vi "Sort Fcurve wfms.vi"(0 "reference in":refnum<class "Fcurve.lvclass">, 1 "Channels In":waveform(dbl)[](array[waveform]), 5 "error in (no error)":errorcluster) -> (7 "Fcurve out":cluster{"X":dbl[], "Y":dbl[]}[](graph), 14 "reference out":refnum<class "Fcurve.lvclass">, 19 "error out":errorcluster)   [LabVIEW 2019, in "Fcurve.lvclass"]
doc: "Sorts wfms into Fcurve. [0] Deflection, [1] Zposition"
uses:
  Fcurve.lvclass
  TDMS_DataHandler_class/property name combo box.ctl
  TDMS_DataHandler_class/TDMS_DataHandler.lvclass
panel:
  out "contact point index out":i32
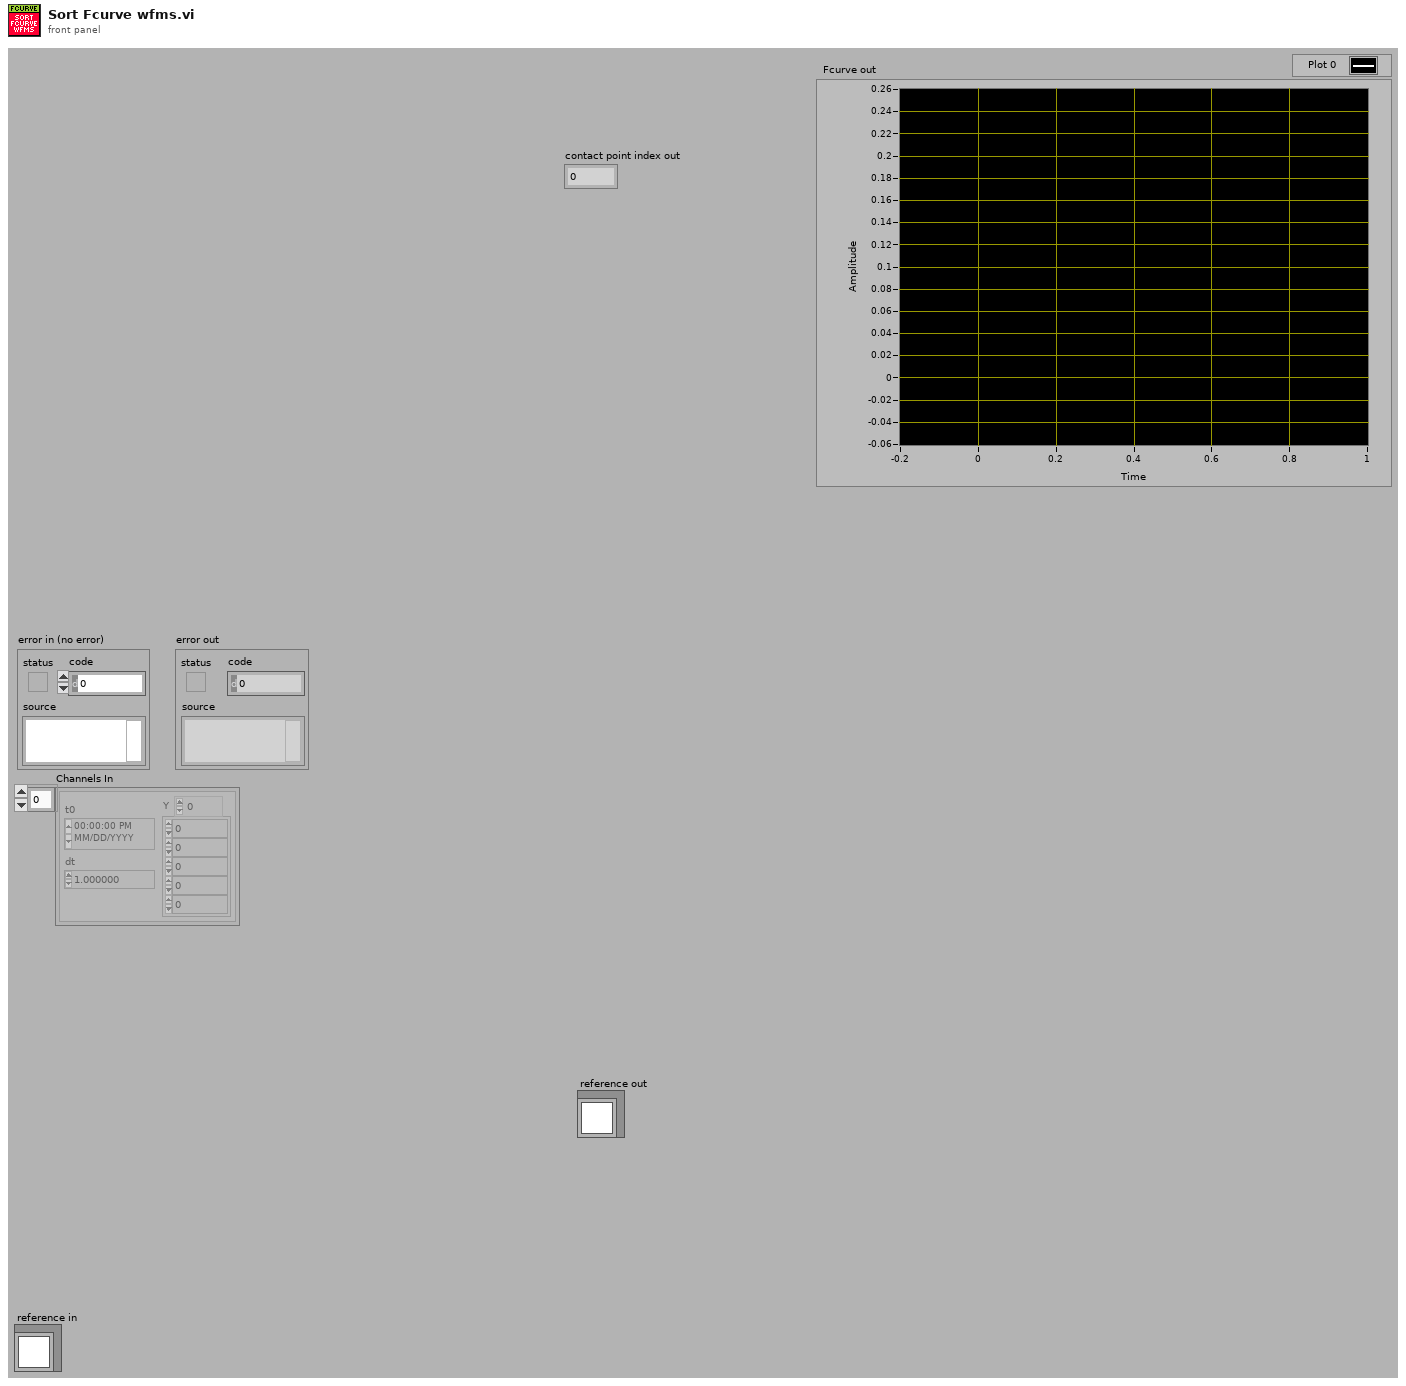
[diagram p1: front panel]
types:
  T1 = typedef "TDMS_DataHandler.lvclass/property name combo box.ctl" = string
  T2 = typedef "Fcurve.lvclass/ObjectAttributes.ctl" = cluster{"MyAttribute":dbl, "Fcurve Metadata":T3, "Contact Spread of dev":dbl, "Tau Delay (ms)":dbl, "Points of contact":dbl, "Def_wfm":cluster{"Max":dbl, "Min":dbl}, "Zpos_wfm":cluster{"Max":dbl, "Min":dbl}, "Contact stat?":bool, "Real AI dt (s)":dbl, "Decimation":cluster{"App":cluster{"Dec":i32, "apply":bool}, "Con":cluster{"Dec":i32, "apply":bool}, "Ret":cluster{"Dec":i32, "apply":bool}}, "Segment def[0]":dbl, "Segment Zpos[0]":dbl, "Raw Datum":waveform(dbl)[], "Group metadata":T4, "M_data obj":refnum<class "metadata.lvclass">, "Channel name(s)":string[], "Segment fcurve data":cluster{"X":dbl[], "Y":dbl[]}[], "Segment duration":cluster{"Start":i32, "Duration":i32}[], "Segment info":T5[], "Segment durations (S)":dbl[], "Segments Maxmin":T7[]}
  T3 = typedef "Fcurve.lvclass/Metadata.ctl" = cluster{"dt (us)":dbl, "Dec Factor":dbl, "Z piezo Sensitivity (nm/V)":dbl, "K (N/m)":dbl, "Sp (V)":dbl, "Contact (ms)":dbl, "Zpos contact":dbl, "Vel_app (nm/s)":dbl, "Vel_ret (nm/s)":dbl, "deltaV (nm)":dbl, "Def_V0 (v)":dbl, "Piezo gain":dbl, "invOLS (nm/V)":dbl}
  T4 = typedef "TDMS_DataHandler.lvclass/Fcurve Meta data.ctl" = cluster{"property names":string[], "property values":variant[]}
  T5 = typedef "Fcurve.lvclass/Fcurve segments --cluster.ctl" = cluster{"type":T6, "nb points":i32, "dec factor":u32, "sampling rate (S/s)":u32}
  T6 = typedef "metadata.lvclass/Segment type--combobox.ctl" = string
  T7 = typedef "Fcurve.lvclass/Segment MaxMin --cluster.ctl" = cluster{"Def":cluster{"max value":dbl, "min value":dbl}, "Zpos":cluster{"max value":dbl, "min value":dbl}}
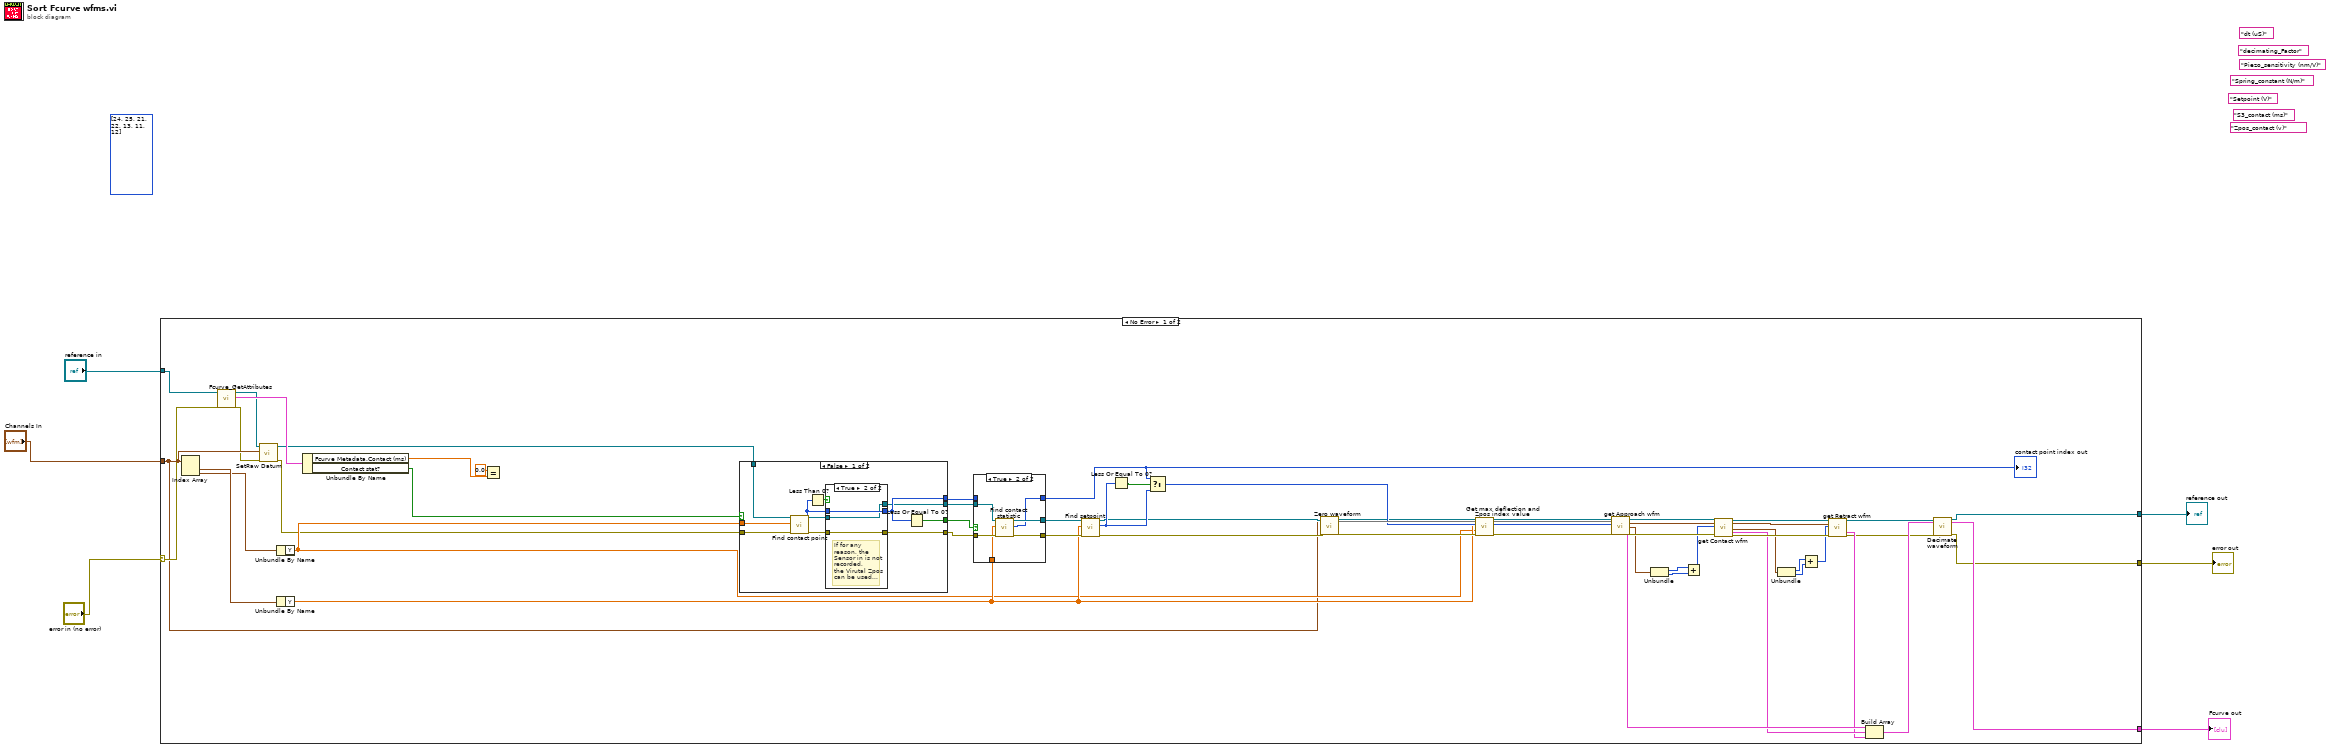
[diagram p0: block diagram]
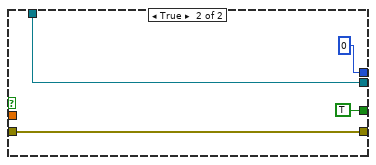
[diagram p3: hidden frame]
diagram:
  (unwired) i32[] [24, 25, 21, 22, 13, 11, 12] ("Array")
  (unwired) T1 "Setpoint (V)" ("Combo Box")
  (unwired) T1 "S3_contact (ms)" ("Combo Box")
  (unwired) T1 "Zpos_contact (v)" ("Combo Box")
  (unwired) T1 "Spring_constant (N/m)" ("Combo Box")
  (unwired) T1 "Piezo_sensitivity (nm/V)" ("Combo Box")
  (unwired) T1 "decimating_Factor" ("Combo Box")
  (unwired) T1 "dt (uS)" ("Combo Box")
  n1 = case shown="No Error" "error in (no error)" {
    selector: "error in (no error)" -> [w26 w92]
    tunnel: "reference in" -> [w59 w93]
    tunnel: [w21 w93] -> w5
    tunnel: [w18 w92] -> w4
    tunnel: [w23 _] -> w2
    tunnel: "Channels In" -> [w11 _]
    frame No Error {
      n2 = Index Array(array=w11) -> (element #1=w25:waveform(dbl), element #2=w24:waveform(dbl))  [unwired: 2 in]
      n3 = call "Fcurve_GetAttributes.vi"("reference in"=w59, "error in (no error)"=w26) -> ("reference out"=w10:refnum<class "Fcurve.lvclass">, "attributes"=w58:T2, "error out"=w8:errorcluster)  [unwired: 14 in, 1 out]
      n4 = call-dynamic "SetRaw Datum.vi"("error in (no error)"=w8, "Raw Datum"=w11, "reference in"=w10) -> ("error out"=w7:errorcluster, "reference out"=w9:refnum<class "Fcurve.lvclass">)  [unwired: 7 in]
      n5 = Unbundle By Name(w24) -> ("Y"=w12:dbl[])
      n6 = Unbundle By Name(w25) -> ("Y"=w13:dbl[])
      n7 = Unbundle By Name(w58) -> ("Fcurve Metadata.Contact (ms)"=w57:dbl, "Contact stat?"=w27:bool)
      n8 = Equal?(x=0.0, y=w57) -> ()  [unwired: 1 out]
      n9 = case shown="False" w27 {
        tunnel: [w64 TRUE] -> w35
        tunnel: [w65 0 ("Zpos index")] -> w60
        tunnel: w9 -> [w72 w79]
        tunnel: w12 -> [w71 _]
        tunnel: w7 -> [w70 w80]
        tunnel: [w68 w80] -> w56
        tunnel: [w62 w79] -> w55
        frame False {
          n10 = call "Find contact point.vi"("reference in"=w72, "Z pos (V)"=w71, "error in (no error)"=w70) -> ("reference out"=w63:refnum<class "Fcurve.lvclass">, "contact index"=w66:i32, "error out"=w67:errorcluster)  [unwired: 14 in]
          n11 = Less Than 0?(x=w66) -> (x < 0?=w69:bool)
          n12 = case shown="True" w69 {
            tunnel: [w75 w78] -> w68
            tunnel: w67 -> [w75 w78]
            tunnel: [w74 w77] -> w65
            tunnel: w66 -> [w74 w77]
            tunnel: w63 -> [w73 w76]
            tunnel: [w73 w76] -> w62
            frame False {
            }
            frame True {
              # "If for any reason, the Sensor in is not recorded,\nthe Virutal Zpos can be used..."
            }
          }
          n13 = Less Or Equal To 0?(x=w65) -> (x <= 0?=w64:bool)
        }
        frame True {
        }
      }
      n14 = case shown="True" w35 {
        tunnel: [w83 w89] -> w54
        tunnel: [w85 w90] -> w43
        tunnel: w60 -> [w85 _]
        tunnel: [w84 w91] -> w53
        tunnel: w56 -> [w83 w88]
        tunnel: w55 -> [w84 w87]
        tunnel: w13 -> [_ w86]
        frame False {
        }
        frame True {
          n15 = call "Find contact statistic.vi"("reference in"=w87, "Deflection (V)"=w86, "error in (no error)"=w88) -> ("reference out"=w91:refnum<class "Fcurve.lvclass">, "contact point index out"=w90:i32, "error out"=w89:errorcluster)  [unwired: 14 in]
        }
      }
      "contact point index out" <- w43
      n16 = call "Find setpoint.vi"("reference in"=w53, "Deflection"=w13, "error in (no error)"=w54) -> ("reference out"=w28:refnum<class "Fcurve.lvclass">, "Setpoint index"=w42:i32, "error out"=w40:errorcluster)  [unwired: 14 in]
      n17 = Less Or Equal To 0?(x=w42) -> (x <= 0?=w44:bool)
      n18 = Select(t=w43, s=w44, f=w42) -> (s? t:f=w39:i32)
      n19 = call-dynamic "Zero waveform.vi"("reference in"=w28, 1:w11, "error in (no error)"=w40) -> ("reference out"=w17:refnum<class "Fcurve.lvclass">, 15:w41, "error out"=w15:errorcluster)  [unwired: 11 in, 3 out]
      n20 = call "Get max deflection and Zpos index value.vi"("reference in"=w17, ">Zpos (V): Sensor IN>"=w12, ">Deflection (V)>"=w13, "error in (no error)"=w15) -> ("reference out"=w16:refnum<class "Fcurve.lvclass">, "error out"=w14:errorcluster)  [unwired: 14 in]
      n21 = call-dynamic "get Approach wfm.vi"("reference in"=w16, "Zeroed (wfms.array)"=w41, 2:w39, "error in (no error)"=w14) -> ("reference out"=w50:refnum<class "Fcurve.lvclass">, "Zeroed (wfms.array) out"=w52:waveform(dbl)[], "Index [start,duration]"=w46:cluster{"Start":i32, "Duration":i32}, "Approach"=w38:cluster{"X":dbl[], "Y":dbl[]}, "error out"=w48:errorcluster)  [unwired: 10 in, 1 out]
      n22 = Unbundle(w46) -> ("Start"=w31:i32, "Duration"=w30:i32)
      n23 = Add(x=w31, y=w30) -> (x+y=w29:i32)
      n24 = call-dynamic "get Contact wfm.vi"("reference in"=w50, ".Zeroed (wfms.array)"=w52, "End Index (approach)"=w29, "error in (no error)"=w48) -> ("reference out"=w49:refnum<class "Fcurve.lvclass">, "Zeroed (wfms.array) out"=w51:waveform(dbl)[], "Contact indices [start,duration]"=w45:cluster{"Start":i32, "Duration":i32}, "Contact"=w37:cluster{"X":dbl[], "Y":dbl[]}, "error out"=w47:errorcluster)  [unwired: 10 in, 1 out]
      n25 = Unbundle(w45) -> ("Start"=w34:i32, "Duration"=w33:i32)
      n26 = Add(x=w34, y=w33) -> (x+y=w32:i32)
      n27 = call-dynamic "get Retract wfm.vi"("reference in"=w49, "Zeroed (wfms.array)"=w51, "End contact (index)"=w32, "error in (no error)"=w47) -> ("reference out"=w22:refnum<class "Fcurve.lvclass">, "Retract"=w36:cluster{"X":dbl[], "Y":dbl[]}, "error out"=w19:errorcluster)  [unwired: 10 in, 3 out]
      n28 = Build Array(w38, w37, w36) -> (w20:cluster{"X":dbl[], "Y":dbl[]}[])
      n29 = call-dynamic "Decimate waveform.vi"("reference in"=w22, 1:w20, "error in (no error)"=w19) -> ("reference out"=w21:refnum<class "Fcurve.lvclass">, "Decimated Fcurve (App,Con,Ret)"=w23:cluster{"X":dbl[], "Y":dbl[]}[], "error out"=w18:errorcluster)  [unwired: 14 in]
    }
    frame Error {
    }
  }
  "error out" <- w4
  "reference out" <- w5
  "Fcurve out" <- w2
